vi "find-path v2.vi"(4 "Start Y":i32, 6 "Start X":i32, 7 "Obstacles":bool[][](array[boolean]), 8 "Destination Y":i16, 9 "Destination X":i16, 10 "Empty Value":dbl, 11 "Wall Value":dbl) -> (2 "Instructions":i32[][](array[numeric]), 3 "appended array":dbl[][](array[numeric]))   [LabVIEW 2015]
uses:
  <vilib>/robotics/Navigation/shared/WorldMap/OccupancyGridWorldMap/NI_Robotics_OccupancyGridWorldMap.lvclass
  <vilib>/robotics/Navigation/NI_Robotics_Navigation .lvlib
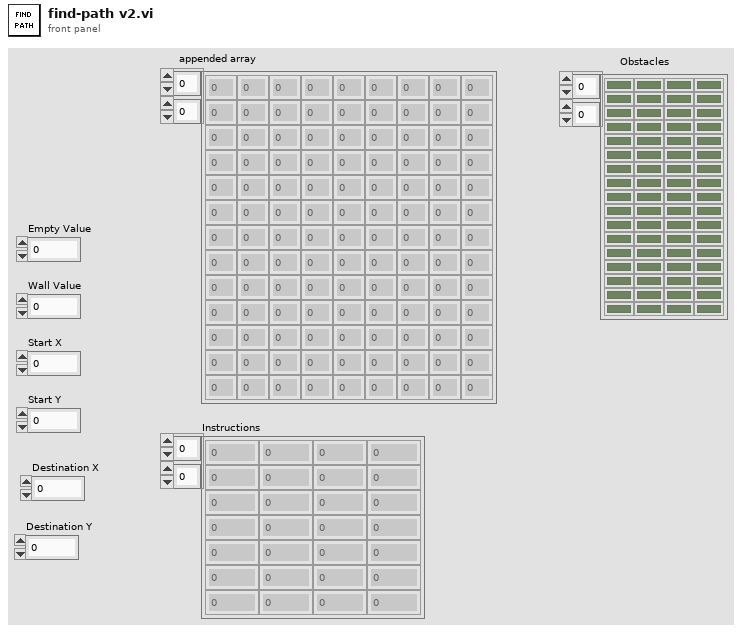
[diagram p1: front panel]
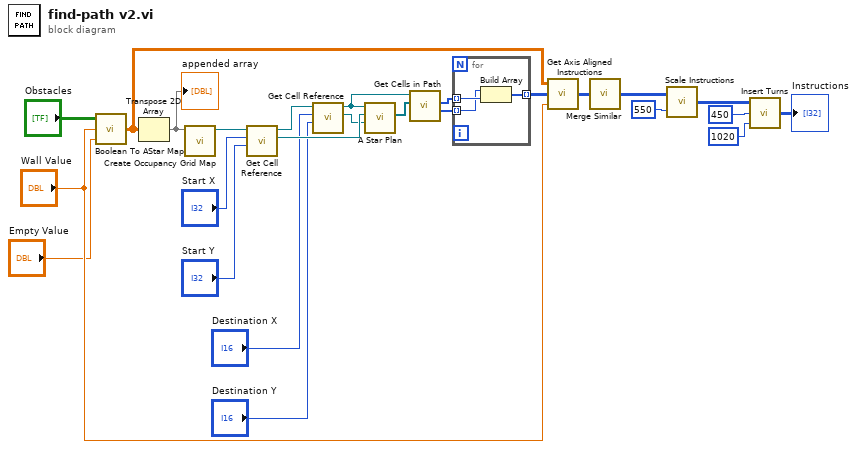
[diagram p0: block diagram]
diagram:
  n1 = call "Boolean To AStar Map.vi"("empty value"="Empty Value", "Wall value"="Wall Value", "Obstacles"="Obstacles") -> ("a star map"=w13:dbl[][])
  n2 = Transpose 2D Array(2D array=w13) -> (transposed array=w14:dbl[][])
  "appended array" <- w14
  n3 = call <vilib>:"Create Occupancy Grid Map.vi"("occupancy grid"=w14) -> ("map reference out"=w15:refnum<data-value>)  [unwired: 9 in, 1 out]
  n4 = call <vilib>:"Get Cell Reference.vi"("y"="Start Y", "x"="Start X", "map reference in"=w15) -> ("cell reference"=w20:refnum<data-value>, "map reference out"=w18:refnum<data-value>)  [unwired: 5 in, 2 out]
  n5 = call <vilib>:"Get Cell Reference.vi"("y"="Destination Y", "x"="Destination X", "map reference in"=w18) -> ("cell reference"=w19:refnum<data-value>, "map reference out"=w22:refnum<data-value>)  [unwired: 5 in, 2 out]
  n6 = call <vilib>:"A Star Plan.vi"("goal reference"=w19, "start reference"=w20, "map reference in"=w22) -> ("path references"=w21:refnum<data-value>[])  [unwired: 5 in, 3 out]
  n7 = call <vilib>:"Get Cells in Path.vi"("path references"=w21, "map reference in"=w22) -> ("y coordinates"=w24:i32[], "x coordinates"=w23:i32[])  [unwired: 6 in, 2 out]
  n8 = for {
    tunnel: w23 -> [w27] mode=indexing
    tunnel: w24 -> [w26] mode=indexing
    tunnel: [w28] -> w7 mode=indexing
    n9 = Build Array(w26, w27) -> (w28:i32[])
  }
  n10 = call "Get Axis Aligned Instructions.vi"("Wall value"="Wall Value", "Key Points"=w7, "obstacles"=w13) -> ("AA Instructions"=w25:i32[][])
  n11 = call "Merge Similar.vi"("AA Instructions"=w25) -> ("Merged Instructions"=w5:i32[][])
  n12 = call "Scale Instructions.vi"("Scale"=i16 550, "Instructions"=w5) -> ("Scaled Instructions"=w4:i32[][])
  n13 = call "Insert Turns.vi"("Sideways Turn Movement"=1020, "Forward Turn Movement"=450, "Merged Instructions"=w4) -> ("Instructions"=→"Instructions":i32[][])
